vi "PPMS_Femto_GUI.vi"() -> ()   [LabVIEW 2010]
uses:
  <userlib>/FEMTO/FEMTO_LUCI-10.lvlib
panel:
  in  "execute!":bool
  in  "stop!":bool
  in  "Choose Amplifier:":u16(ring) items=["1 - DDPCA", "2 - DDPCA", "3 - DDPCA", "4 - DLPVA"]
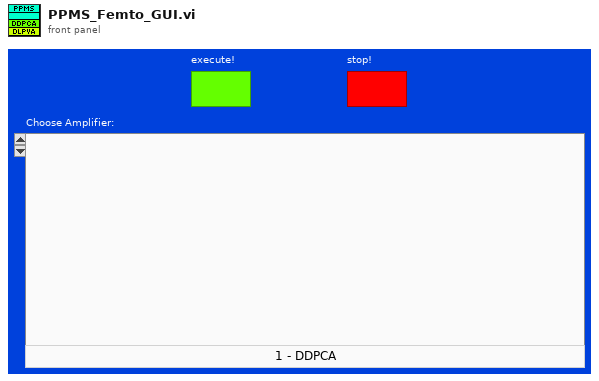
[diagram p1: front panel]
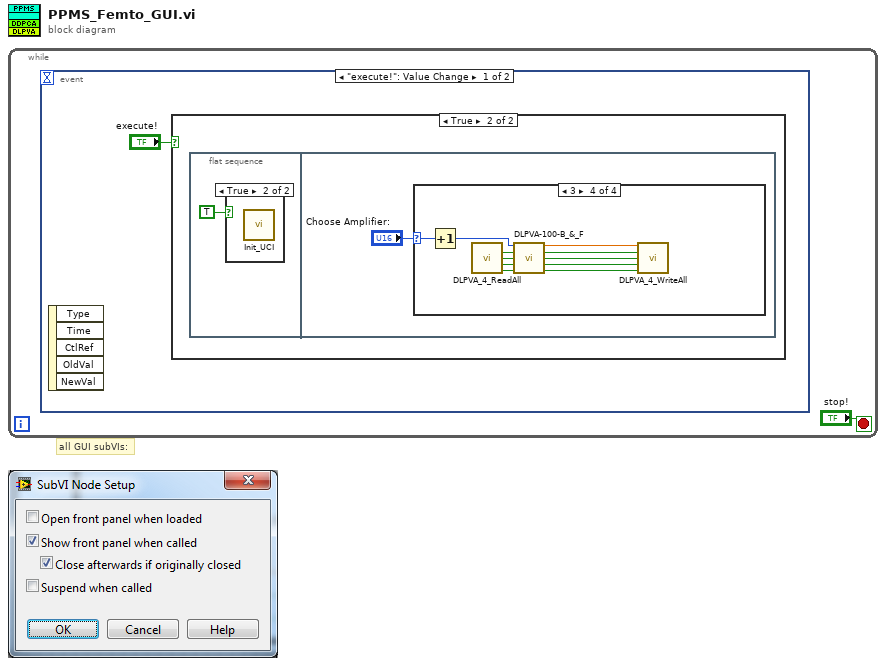
[diagram p0: block diagram]
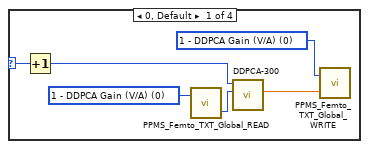
[diagram p4: hidden frame]
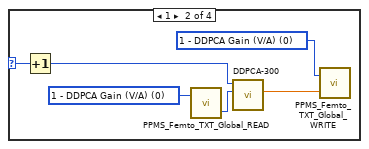
[diagram p5: hidden frame]
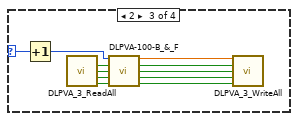
[diagram p6: hidden frame]
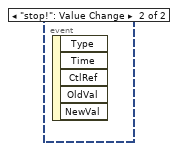
[diagram p7: hidden frame]
diagram:
  # "all GUI subVIs:"
  n1 = while {
    stop <- "stop!" stop-if-true
    n2 = event shown="[0] \"execute!\": Value Change" {
      selector: _ -> [_ _]
      dyn-events: _ -> [_ _]
      timeout: _ -> [_ _]
      event "execute!": Value Change {
        n3 = event-data() -> ()  [unwired: 1 in, 5 out]
        n4 = case shown="True" "execute!" {
          frame False {
          }
          frame True {
            n5 = flat-sequence {
              frame #0 {
                n6 = case shown="True" TRUE ("initialize?") {
                  frame False {
                  }
                  frame True {
                    n7 = call <userlib>:"Init_UCI.vi"() -> ()  [unwired: 10 in, 2 out]
                  }
                }
              }
              frame #1 {
                n8 = case shown="3" "Choose Amplifier:" {
                  selector: "Choose Amplifier:" -> [w10 w16 w27 w38]
                  frame 0, Default {
                    w7 = u16 0 items=["1 - DDPCA Gain (V/A)", "2 - DDPCA Gain (V/A)", "3 - DLPVA Gain (dB)", "3 - Gain 1", "3 - Gain 2", "3 - AC/DC coupling", "3 - filter", "4 - DLPVA Gain (dB)", "4 - Gain 1", "4 - Gain 2", "4 - AC/DC coupling", "4 - filter"] ("Property")
                    w6 = u16 0 items=["1 - DDPCA Gain (V/A)", "2 - DDPCA Gain (V/A)", "3 - DLPVA Gain (dB)", "3 - Gain 1", "3 - Gain 2", "3 - AC/DC coupling", "3 - filter", "4 - DLPVA Gain (dB)", "4 - Gain 1", "4 - Gain 2", "4 - AC/DC coupling", "4 - filter"] ("Property")
                    n9 = Increment(x=w10) -> (x+1=w9:u16)
                    n10 = call "PPMS_Femto_TXT_Global_READ.vi"("Property"=w6) -> ("Value"=w5:i32)  [unwired: 1 in, 1 out]
                    n11 = call "DDPCA-300.vi"("Gain (V/A)"=w5, "Index"=w9) -> ("Gain (V/A)"=w8:dbl)  [unwired: 9 in]
                    n12 = call "PPMS_Femto_TXT_Global_WRITE.vi"("Value"=w8, "Property"=w7) -> ()  [unwired: 2 in]
                  }
                  frame 1 {
                    w14 = u16 0 items=["1 - DDPCA Gain (V/A)", "2 - DDPCA Gain (V/A)", "3 - DLPVA Gain (dB)", "3 - Gain 1", "3 - Gain 2", "3 - AC/DC coupling", "3 - filter", "4 - DLPVA Gain (dB)", "4 - Gain 1", "4 - Gain 2", "4 - AC/DC coupling", "4 - filter"] ("Property")
                    w11 = u16 0 items=["1 - DDPCA Gain (V/A)", "2 - DDPCA Gain (V/A)", "3 - DLPVA Gain (dB)", "3 - Gain 1", "3 - Gain 2", "3 - AC/DC coupling", "3 - filter", "4 - DLPVA Gain (dB)", "4 - Gain 1", "4 - Gain 2", "4 - AC/DC coupling", "4 - filter"] ("Property")
                    n13 = Increment(x=w16) -> (x+1=w15:u16)
                    n14 = call "PPMS_Femto_TXT_Global_READ.vi"("Property"=w11) -> ("Value"=w12:i32)  [unwired: 1 in, 1 out]
                    n15 = call "DDPCA-300.vi"("Gain (V/A)"=w12, "Index"=w15) -> ("Gain (V/A)"=w13:dbl)  [unwired: 9 in]
                    n16 = call "PPMS_Femto_TXT_Global_WRITE.vi"("Value"=w13, "Property"=w14) -> ()  [unwired: 2 in]
                  }
                  frame 2 {
                    n17 = Increment(x=w27) -> (x+1=w26:u16)
                    n18 = call "DLPVA_3_ReadAll.vi"() -> ("gain 1"=w18:bool, "gain 2"=w17:bool, "coupling"=w25:bool, "filter"=w24:bool)  [unwired: 12 in]
                    n19 = call "DLPVA-100-B_&_F.vi"("Index"=w26, "Gain_1 i"=w18, "Gain_2 i"=w17, "AC/DC"=w25, "Filter"=w24) -> ("Gain (dB)"=w20:dbl, "Gain_1o"=w23:bool, "Gain_2 o"=w22:bool, "AC/DC o"=w21:bool, "Filter o"=w19:bool)  [unwired: 6 in]
                    n20 = call "DLPVA_3_WriteAll.vi"("Gain (dB)"=w20, "Gain_1o"=w23, "Gain_2 o"=w22, "AC/DC o"=w21, "Filter o"=w19) -> ()  [unwired: 11 in]
                  }
                  frame 3 {
                    n21 = Increment(x=w38) -> (x+1=w37:u16)
                    n22 = call "DLPVA_4_ReadAll.vi"() -> ("gain 1"=w36:bool, "gain 2"=w35:bool, "coupling"=w34:bool, "filter"=w33:bool)  [unwired: 12 in]
                    n23 = call "DLPVA-100-B_&_F.vi"("Index"=w37, "Gain_1 i"=w36, "Gain_2 i"=w35, "AC/DC"=w34, "Filter"=w33) -> ("Gain (dB)"=w32:dbl, "Gain_1o"=w31:bool, "Gain_2 o"=w30:bool, "AC/DC o"=w29:bool, "Filter o"=w28:bool)  [unwired: 6 in]
                    n24 = call "DLPVA_4_WriteAll.vi"("Gain (dB)"=w32, "Gain_1o"=w31, "Gain_2 o"=w30, "AC/DC o"=w29, "Filter o"=w28) -> ()  [unwired: 11 in]
                  }
                }
              }
            }
          }
        }
      }
      event "stop!": Value Change {
        n25 = event-data() -> ()  [unwired: 1 in, 5 out]
      }
    }
  }
